vi "Number of Active Paths.vi"(11 "Active Paths":T1=[TRUE, TRUE, TRUE, TRUE]) -> (3 "Number of Active Paths":i32)   [LabVIEW 2011]
uses:
  UI typedefs/Active Paths.ctl
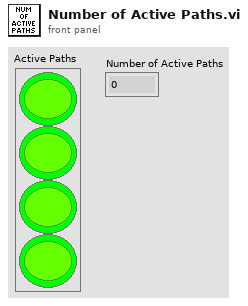
[diagram p1: front panel]
types:
  T1 = typedef "Active Paths.ctl" = bool[]
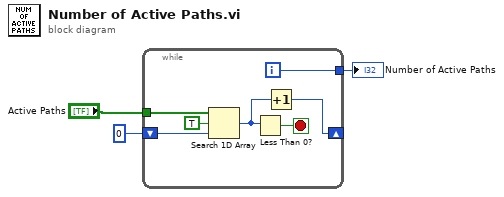
[diagram p0: block diagram]
diagram:
  n1 = while {
    tunnel: "Active Paths" -> [w9]
    shift-right: [w5] -> _
    shift-left: 0 ("start index (0)") -> [w8]
    tunnel: [w4] -> w2
    i -> [w4]
    stop <- w6 stop-if-true
    n2 = Search 1D Array(1D array=w9, element=TRUE, start index (0)=w8) -> (index of element=w7:i32)
    n3 = Less Than 0?(x=w7) -> (x < 0?=w6:bool)
    n4 = Increment(x=w7) -> (x+1=w5:i32)
  }
  "Number of Active Paths" <- w2
